vi "Calc_Portfolio_at_Date.vi"(0 "Portfolio en entrée":refnum<class "Portfolio.lvclass"> caption="DNL_LabVIEW Object in", 5 "Date":timestamp, 11 "error in (no error)":errorcluster caption="entrée d'erreur (pas d'erreur)") -> (3 "Change-couleurs":u32[](array[numeric]), 4 "Portfolio en sortie":refnum<class "Portfolio.lvclass"> caption="DNL_LabVIEW Object out", 6 "Qtés":dbl[](array[numeric]), 8 "Valo-couleurs":u32[](array[numeric]), 10 "Stocks":refnum<class "Stock.lvclass">[](array[class]), 12 "Montant investi":dbl, 13 "Done ?":bool, 14 "Tableau":string[][](array[string]), 15 "error out":errorcluster caption="sortie d'erreur")   [LabVIEW 2012, in "Portfolio.lvclass"]
uses:
  Portfolio.lvclass
  Stock/Stock.lvclass
  Portfolio.lvclass/Portfolio.ctl
  Stocks Manager/Stock Manager Action.ctl
  Stock/Stock.lvclass/Stock.ctl
  Exchanges/Exchanges.lvclass
  Operations/Operations.lvclass
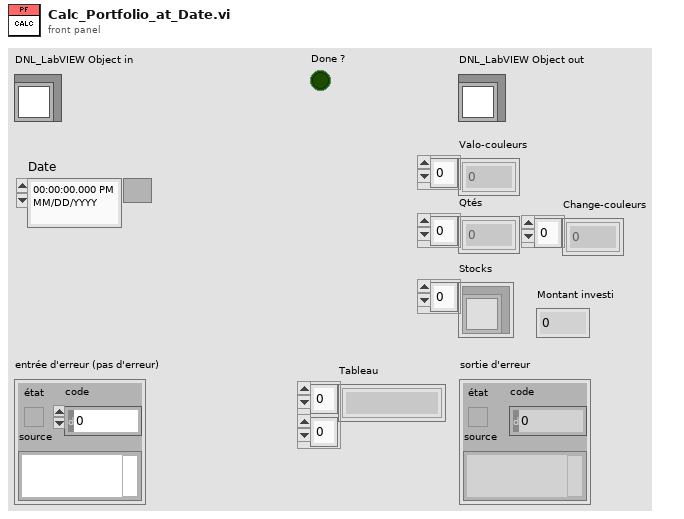
[diagram p1: front panel]
types:
  T1 = typedef "Stock Manager Action.ctl" = enum16{"Get_Stocks", "Load_Stocks", "Find_Stock_From_ISIN", "Find_Stock_From_Label", "Find_Stock_From_Symbol"}
  T2 = typedef "Operation Parameters.ctl" = cluster{"Date":timestamp, "Operation Type":T3, "Amount":dbl, "Comment":string, "Currency":T4}
  T3 = typedef "Operation Type Enum.ctl" = enum16{"Coupons", "Dépot", "Retrait", "Intérêts", "Taxe"}
  T4 = typedef "Currencies.ctl" = enum16{"Euro", "Dollar", "Yen", "RIM", "CHF"}
  T5 = typedef "Exchange Parameters.ctl" = cluster{"Date":timestamp, "Exchange Type":T6, "ISIN":string, "Label":string, "Price":dbl, "Qty":dbl, "Currency":T4, "Tax":dbl, "Comment":string, "PRU":dbl}
  T6 = typedef "Exchange.lvclass/Exchange Type Enum.ctl" = enum16{"ACHAT", "VENTE"}
  T7 = typedef "Stock.lvclass/Stock Parameters.ctl" = cluster{"Label":string, "Symbol":string, "Dividend":dbl, "Currency":T4, "ISIN":string, "Symbol_Suffix":string, "Last Price":dbl, "Dividend-Date":string, "Change (%)":dbl, "Objective":dbl, "Stop":dbl}
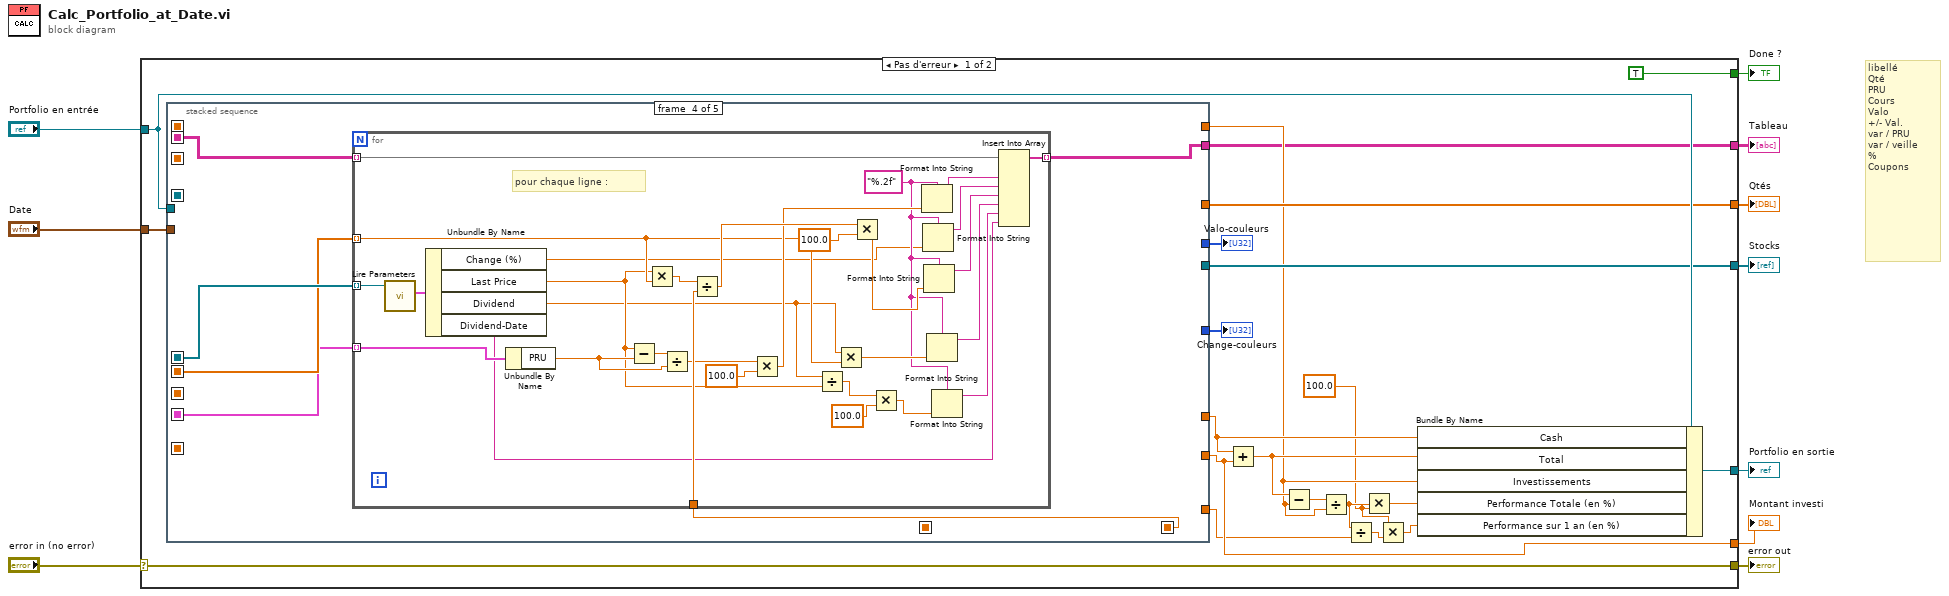
[diagram p0: block diagram]
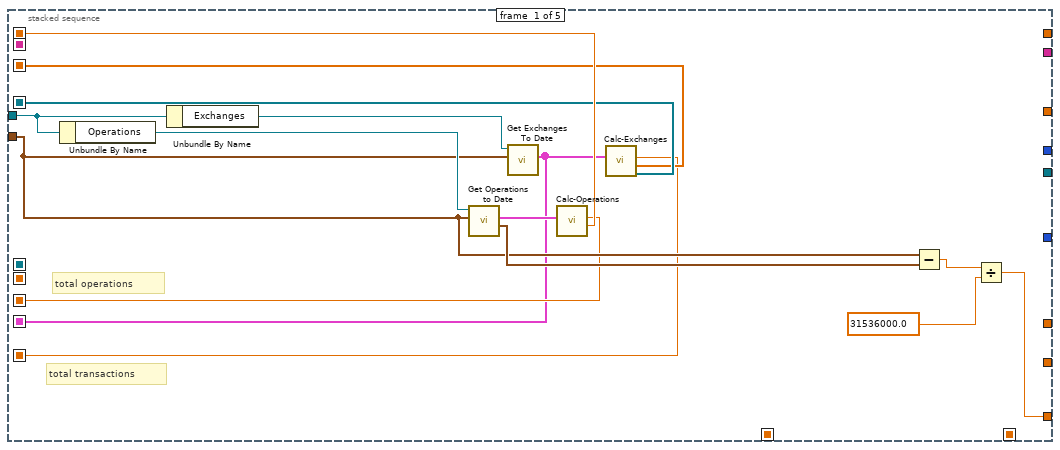
[diagram p2: hidden frame]
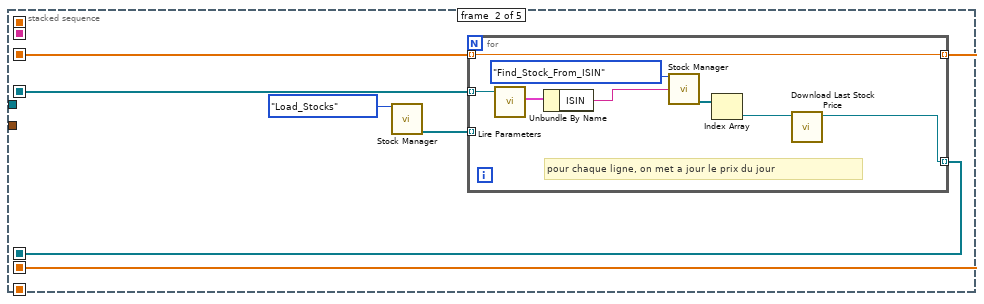
[diagram p3: hidden frame]
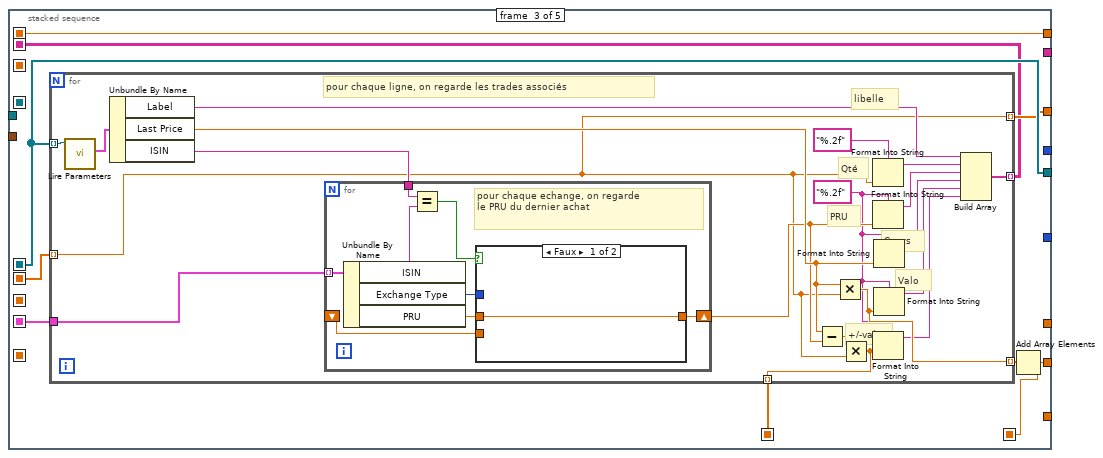
[diagram p4: hidden frame]
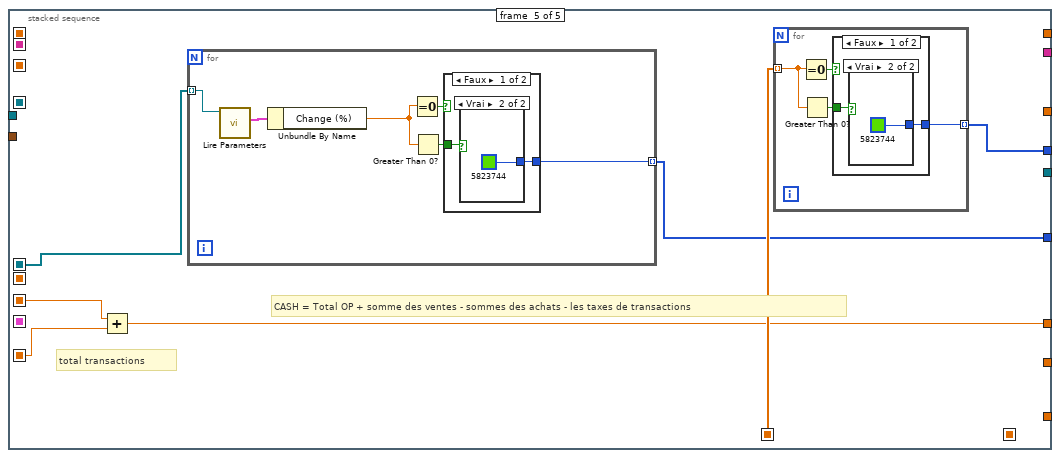
[diagram p7: hidden frame]
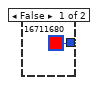
[diagram p8: hidden frame]
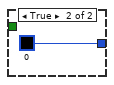
[diagram p9: hidden frame]
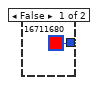
[diagram p10: hidden frame]
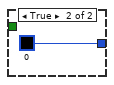
[diagram p11: hidden frame]
diagram:
  # "libellé\nQté\nPRU\nCours\nValo\n+/- Val.\nvar / PRU\nvar / veille\n%\nCoupons"
  n1 = case shown="Pas d'erreur" "error in (no error)" {
    selector: "error in (no error)" -> [w31 w168]
    tunnel: [w31 w168] -> w9
    tunnel: [w29 w167] -> w7
    tunnel: "Portfolio en entrée" -> [w30 w167]
    tunnel: "Date" -> [w28 _]
    tunnel: [w27 _] -> w5
    tunnel: [w19 _] -> w4
    tunnel: [w26 _] -> w3
    tunnel: [w21 _] -> w2
    tunnel: [TRUE _] -> w1
    frame No Error {
      w14 = 100.0 ("y")
      n2 = stacked-sequence {
        seq-local: [w36 _ _ _ _] -> [_ _ _ _ w143]
        seq-local: [w33 _ _ _ _] -> [_ _ _ _ w144]
        seq-local: [w32 _ _ _ _] -> [_ _ w67 w104 _]
        seq-local: [w35 _ _ _ _] -> [_ w47 _ _ _]
        seq-local: [w34 _ _ _ _] -> [_ w48 _ _ _]
        seq-local: [_ w52 _ _ _] -> [_ _ w68 w107 w141]
        seq-local: [_ w51 _ _ _] -> [_ _ w69 w105 _]
        seq-local: [w37 _ _ _ _] -> [_ _ w64 _ _]
        seq-local: [_ _ w63 _ _] -> [_ _ _ _ w146]
        seq-local: [_ _ w62 _ _] -> [_ _ _ w109 _]
        seq-local: [_ _ w61 _ _] -> [_ _ _ w108 _]
        tunnel: w30 -> [w40 _ _ _ _]
        tunnel: [_ _ _ _ w142] -> w25
        tunnel: w28 -> [w39 _ _ _ _]
        tunnel: [_ _ w68 _ _] -> w27
        tunnel: [_ _ w66 _ _] -> w26
        tunnel: [_ _ w61 _ _] -> w21
        tunnel: [_ _ w64 _ _] -> w22
        tunnel: [_ _ _ _ w145] -> w20
        tunnel: [_ _ _ w106 _] -> w19
        tunnel: [w44 _ _ _ _] -> w15
        tunnel: [_ _ _ _ w140] -> w11
        frame #0 {
          # "total operations"
          # "total transactions"
          n3 = Unbundle By Name(w40) -> ("Operations"=w43:refnum<class "Operations.lvclass">)
          n4 = Unbundle By Name(w40) -> ("Exchanges"=w41:refnum<class "Exchanges.lvclass">)
          n5 = call "Get Operations to Date.vi"("Date"=w39, "Operations en entrée"=w43) -> ("Min Date"=w42:timestamp, "Operations Found at Date"=w38:T2[])  [unwired: 6 in, 2 out]
          n6 = call "Get Exchanges To Date.vi"("Date"=w39, "Exchanges en entrée"=w41) -> ("Exchanges to Date"=w32:T5[])  [unwired: 6 in, 3 out]
          n7 = call "Calc-Operations.vi"("Operations"=w38) -> ("Investissement"=w37:dbl, "Total OP"=w36:dbl)  [unwired: 9 in]
          n8 = call "Calc-Exchanges.vi"("Exchanges"=w32) -> ("Lignes"=w35:refnum<class "Stock.lvclass">[], "Qtés restante par ligne"=w34:dbl[], "Total"=w33:dbl)  [unwired: 8 in]
          n9 = Subtract(x=w39, y=w42) -> (x-y=w46:dbl)
          n10 = Divide(x=w46, y=31536000.0) -> (x/y=w44:dbl)
        }
        frame #1 {
          n11 = call "Stock Manager.vi"("Stock Manager Action"=Stock_Manager_Action."Load_Stocks") -> ("Stocks Found"=w50:refnum<class "Stock.lvclass">[])  [unwired: 12 in, 2 out]
          n12 = for {
            tunnel: w48 -> [w54] mode=indexing
            tunnel: w47 -> [w59] mode=indexing
            tunnel: [w53] -> w52 mode=indexing
            tunnel: [w54] -> w51 mode=indexing
            tunnel: w50 -> [_] mode=indexing
            # "pour chaque ligne, on met a jour le prix du jour"
            n13 = call "Lire Parameters.vi"("Stock en entrée"=w59) -> ("Parameters"=w58:T7)  [unwired: 9 in, 1 out]
            n14 = Unbundle By Name(w58) -> ("ISIN"=w57:string)
            n15 = call "Stock Manager.vi"("Stock Manager Action"=Stock_Manager_Action."Find_Stock_From_ISIN", "String to find (ISIN,Label,Symbol)"=w57) -> ("Stocks Found"=w56:refnum<class "Stock.lvclass">[])  [unwired: 11 in, 2 out]
            n16 = Index Array(array=w56) -> (element=w55:refnum<class "Stock.lvclass">)  [unwired: 1 in]
            n17 = call "Download Last Stock Price.vi"("Share en entrée"=w55) -> ("Share en sortie"=w53:refnum<class "Stock.lvclass">)  [unwired: 7 in, 3 out]
          }
        }
        frame #2 {
          n18 = for {
            tunnel: w68 -> [w88] mode=indexing
            tunnel: [w86] -> w62 mode=indexing
            tunnel: w69 -> [w74] mode=indexing
            tunnel: w67 -> [w79]
            tunnel: [w74] -> w66 mode=indexing
            tunnel: [w78] -> w65 mode=indexing
            tunnel: [w72] -> w63 mode=indexing
            w73 = "%.2f" ("chaîne de format")
            # "+/-val"
            # "Valo"
            # "Cours"
            # "PRU"
            # "Qté"
            # "libelle"
            # "pour chaque ligne, on regarde les trades associés"
            n19 = call "Lire Parameters.vi"("Stock en entrée"=w88) -> ("Parameters"=w87:T7)  [unwired: 9 in, 1 out]
            n20 = Unbundle By Name(w87) -> ("Label"=w82:string, "Last Price"=w77:dbl, "ISIN"=w83:string)
            n21 = for {
              tunnel: w79 -> [w96] mode=indexing
              tunnel: w83 -> [w95]
              shift-right: [w90] -> w76
              shift-left: _ -> [w89]
              # "pour chaque echange, on regarde\nle PRU du dernier achat"
              n22 = Unbundle By Name(w96) -> ("ISIN"=w94:string, "Exchange Type"=w92:T6, "PRU"=w91:dbl)
              n23 = Equal?(x=w95, y=w94) -> (x = y?=w93:bool)
              n24 = case shown="Faux" w93 {
                tunnel: w92 -> [_ w101]
                tunnel: w91 -> [_ w100]
                tunnel: [w97 w99] -> w90
                tunnel: w89 -> [w97 w98]
                frame False {
                }
                frame True {
                  n25 = case shown="\"ACHAT\"" w101 {
                    tunnel: w100 -> [w102 _]
                    tunnel: [w102 w103] -> w99
                    tunnel: w98 -> [_ w103]
                    frame "ACHAT" {
                    }
                    frame "VENTE", Default {
                    }
                  }
                }
              }
            }
            n26 = Subtract(x=w77, y=w76) -> (x-y=w75:dbl)
            n27 = Multiply(x=w77, y=w74) -> (x*y=w78:dbl)
            n28 = Multiply(x=w75, y=w74) -> (x*y=w72:dbl)
            n29 = Format Into String(format string="%.2f" ("chaîne de format"), w74) -> (resulting string=w85:string)  [unwired: 2 in, 1 out]
            n30 = Format Into String(format string=w73, w76) -> (resulting string=w81:string)  [unwired: 2 in, 1 out]
            n31 = Format Into String(format string=w73, w72) -> (resulting string=w71:string)  [unwired: 2 in, 1 out]
            n32 = Format Into String(format string=w73, w77) -> (resulting string=w84:string)  [unwired: 2 in, 1 out]
            n33 = Format Into String(format string=w73, w78) -> (resulting string=w80:string)  [unwired: 2 in, 1 out]
            n34 = Build Array(w82, w85, w81, w84, w80, w71) -> (w86:string[])
          }
          n35 = Add Array Elements(numeric array=w65) -> (sum=w61:dbl)
        }
        frame #3 {
          n36 = for {
            tunnel: w109 -> [w139] mode=indexing
            tunnel: w108 -> [w134]
            tunnel: w107 -> [w138] mode=indexing
            tunnel: [w136] -> w106 mode=indexing
            tunnel: w105 -> [w117] mode=indexing
            tunnel: w104 -> [w131] mode=indexing
            w119 = "%.2f" ("chaîne de format")
            # "pour chaque ligne :"
            n37 = call "Lire Parameters.vi"("Stock en entrée"=w138) -> ("Parameters"=w137:T7)  [unwired: 9 in, 1 out]
            n38 = Unbundle By Name(w137) -> ("Change (%)"=w110:dbl, "Last Price"=w116:dbl, "Dividend"=w112:dbl, "Dividend-Date"=w111:string)
            n39 = Unbundle By Name(w131) -> ("PRU"=w129:dbl)
            n40 = Subtract(x=w116, y=w129) -> (x-y=w130:dbl)
            n41 = Multiply(x=w116, y=w117) -> (x*y=w135:dbl)
            n42 = Divide(x=w130, y=w129) -> (x/y=w128:dbl)
            n43 = Divide(x=w135, y=w134) -> (x/y=w133:dbl)
            n44 = Multiply(x=w128, y=100.0) -> (x*y=w124:dbl)
            n45 = Divide(x=w112, y=w116) -> (x/y=w115:dbl)
            n46 = Multiply(x=w112, y=w117) -> (x*y=w120:dbl)
            n47 = Multiply(x=w133, y=100.0) -> (x*y=w123:dbl)
            n48 = Multiply(x=w115, y=100.0) -> (x*y=w113:dbl)
            n49 = Format Into String(format string=w119, w124) -> (resulting string=w126:string)  [unwired: 2 in, 1 out]
            n50 = Format Into String(format string=w119, w110) -> (resulting string=w125:string)  [unwired: 2 in, 1 out]
            n51 = Format Into String(format string=w119, w123) -> (resulting string=w122:string)  [unwired: 2 in, 1 out]
            n52 = Format Into String(format string=w119, w120) -> (resulting string=w121:string)  [unwired: 2 in, 1 out]
            n53 = Format Into String(format string=w119, w113) -> (resulting string=w118:string)  [unwired: 2 in, 1 out]
            n54 = Insert Into Array(array=w139, new element #1=w126, new element #2=w125, new element #3=w122, new element #4=w121, new element #5=w118, new element #6=w111) -> (w136:string[])  [unwired: 1 in]
          }
        }
        frame #4 {
          # "total transactions"
          # "CASH = Total OP + somme des ventes - sommes des achats - les taxes de transactions"
          n55 = Add(x=w143, y=w144) -> (x+y=w142:dbl)
          n56 = for {
            tunnel: w141 -> [w151] mode=indexing
            tunnel: [w147] -> w140 mode=indexing
            n57 = call "Lire Parameters.vi"("Stock en entrée"=w151) -> ("Parameters"=w152:T7)  [unwired: 9 in, 1 out]
            n58 = Unbundle By Name(w152) -> ("Change (%)"=w148:dbl)
            n59 = Equal To 0?(x=w148) -> (x = 0?=w150:bool)
            n60 = Greater Than 0?(x=w148) -> (x > 0?=w149:bool)
            n61 = case shown="Faux" w150 {
              tunnel: [w153 u32 0 ("Color")] -> w147
              tunnel: w149 -> [w154 _]
              frame False {
                n62 = case shown="Vrai" w154 {
                  tunnel: [u32 16711680 ("Color") u32 5823744 ("Color")] -> w153
                  frame False {
                  }
                  frame True {
                  }
                }
              }
              frame True {
              }
            }
          }
          n63 = for {
            tunnel: w146 -> [w159] mode=indexing
            tunnel: [w160] -> w145 mode=indexing
            n64 = Equal To 0?(x=w159) -> (x = 0?=w161:bool)
            n65 = Greater Than 0?(x=w159) -> (x > 0?=w158:bool)
            n66 = case shown="Faux" w161 {
              tunnel: [w162 u32 0 ("Color")] -> w160
              tunnel: w158 -> [w163 _]
              frame False {
                n67 = case shown="Vrai" w163 {
                  tunnel: [u32 16711680 ("Color") u32 5823744 ("Color")] -> w162
                  frame False {
                  }
                  frame True {
                  }
                }
              }
              frame True {
              }
            }
          }
        }
      }
      "Valo-couleurs" <- w20
      "Change-couleurs" <- w11
      n68 = Add(x=w25, y=w21) -> (x+y=w24:dbl)
      n69 = Subtract(x=w24, y=w22) -> (x-y=w23:dbl)
      n70 = Divide(x=w23, y=w22) -> (x/y=w16:dbl)
      n71 = Divide(x=w16, y=w15) -> (x/y=w13:dbl)
      n72 = Multiply(x=w16, y=w14) -> (x*y=w17:dbl)
      n73 = Multiply(x=w14, y=w13) -> (x*y=w12:dbl)
      n74 = Bundle By Name(cluster=w30, "Cash"=w25, "Total"=w24, "Investissements"=w22, "Performance Totale (en %)"=w17, "Performance sur 1 an (en %)"=w12) -> (w29:refnum<class "Portfolio.lvclass">)
    }
    frame Error {
    }
  }
  "error out" <- w9
  "Portfolio en sortie" <- w7
  "Stocks" <- w5
  "Qtés" <- w3
  "Tableau" <- w4
  "Montant investi" <- w2
  "Done ?" <- w1
